vi "impedenzimetro.vi"() -> ()   [LabVIEW 2018]
uses:
  <vilib>/Analysis/4window.llb/windowTd.ctl
  <vilib>/Analysis/1siggen.llb/Ramp Pattern by Samples.vi
  <vilib>/DAQmx/write.llb/DAQmx Write (Analog Wfm 1Chan NSamp).vi
  <vilib>/DAQmx/create/channels.llb/DAQmx Create Channel (AO-Voltage-Basic).vi
  <vilib>/DAQmx/configure/timing.llb/DAQmx Timing (Sample Clock).vi
  <vilib>/DAQmx/miscellaneous.llb/DAQmx Fill In Error Info.vi
  <vilib>/measure/maspectr.llb/FFT Spectrum (Mag-Phase) for N Chan.vi
  <vilib>/DAQmx/read.llb/DAQmx Read (Analog 1D Wfm NChan NSamp).vi
  <resource>/objmgr/daqmx.rc
  <vilib>/measure/NI_MAPro.lvlib
  <vilib>/measure/NI_MABase.lvlib
  <vilib>/Analysis/NI_AALBase.lvlib
  <vilib>/Analysis/NI_AALPro.lvlib
panel:
  out "Zx":cdb=3019.4604118764787-15314.276810560117i
  in  "window":T1 items=["Rectangle"=0, "Hanning"=1, "Hamming"=2, "Blackman-Harris"=3, "Exact Blackman"=4, "Blackman"=5, "Flat Top"=6, "4 Term B-Harris "=7, "7 Term B-Harris"=8, "Low Sidelobe"=9, "Blackman Nuttall"=11, "Triangle"=30, "Bartlett-Hanning"=31, "Bohman"=32, "Parzen"=33, "Welch"=34, "Kaiser"=60, "Dolph-Chebyshev"=61, "Gaussian"=62]
  in  "amplitude[V]":dbl=10.0 format="%0.2p"
  in  "end[Hz]":dbl=1000.0 format="%0.2f"
  in  "start[Hz]":dbl=500.0 format="%0.2f"
  in  "samples":i32=10
  in  "Number of Samples":i32=20000
  in  "Sample Rate in[Hz]":dbl=200000.0 format="%#_13g"
  out "C[Farad]":dbl=1.039258628145917e-08 format="%#_6p"
  out "R[Ohm]":dbl=3019.4604118764787
  in  "R Shunt[Ohm]":dbl=300.0
  out "input":waveform(dbl)[](graph)=[{"t0"=timestamp(3731482242.5200343 s since 1904-01-01), "dt"=4.999999999999959e-06, "Y"=array[20000 elements], "attributes"=variant("NI_ChannelName"=variant(string "PXIe_NI6341/ai0"), "NI_UnitDescription"=variant(string "Volts"))}, {"t0"=timestamp(3731482242.520037 s since 1904-01-01), "dt"=4.999999999999959e-06, "Y"=array[20000 elements], "attributes"=variant("NI_ChannelName"=variant(string "PXIe_NI6341/ai1"), "NI_UnitDescription"=variant(string "Volts"))}]
  in  "Max Voltage in":dbl=10.0
  in  "Min Voltage out":dbl=-10.0
  in  "Input":tag="PXIe_NI6341/ai0:1"
  in  "Sample Rate out[Hz]":dbl=200000.0
  in  "Max Voltage out":dbl=10.0
  in  "Min Voltage out":dbl=-10.0
  out "Actual Sample Rate":dbl=200000.0 format="%0.2f"
  in  "Output":tag="PXIe_NI6341/ao0"
  in  "Configurazione scelta":string(combo)="serie"
  # "GENERAZIONE"
  # "CALCOLO DELLE COMPONENTI"
  # "ACQUISIZIONE"
  # "FREQUENZE"
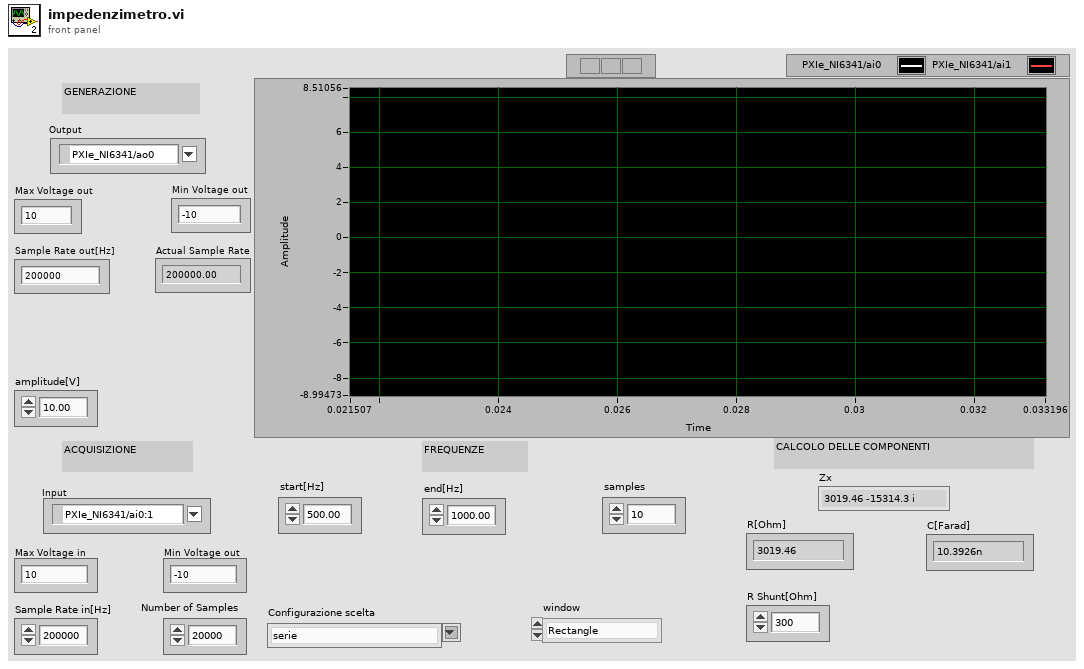
[diagram p1: front panel]
types:
  T1 = typedef "NI_AALPro.lvlib/windowTd.ctl" = u32
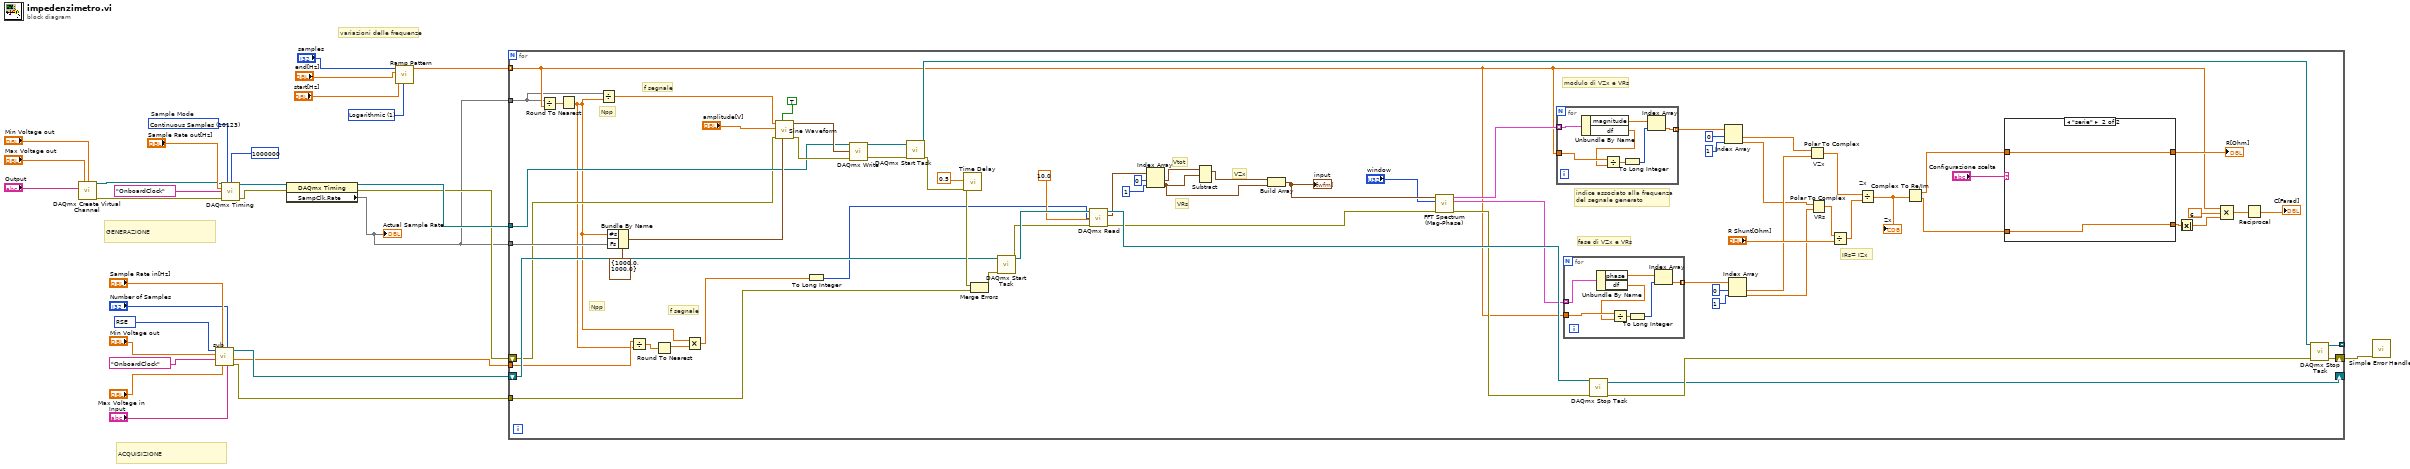
[diagram p0: block diagram]
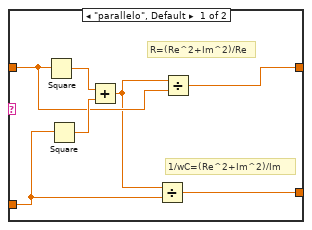
[diagram p2: hidden frame]
diagram:
  w3 = 10083 items=["default"=-1, "RSE"=10083, "NRSE"=10078, "Differential"=10106, "Pseudodifferential"=12529] ("Terminal Configuration")
  w9 = u16 1 items=["Linear", "Logarithmic"] ("type")
  w18 = 10123 items=["Finite Samples"=10178, "Continuous Samples"=10123, "Hardware Timed Single Point"=12522]  # Sample Mode
  # "ACQUISIZIONE"
  # "variazioni delle frequenze"
  # "GENERAZIONE"
  n1 = call-poly <vilib>:"DAQmx Create Virtual Channel.vi"("maximum value"="Max Voltage out", "minimum value"="Min Voltage out", "physical channels"="Output") -> ("task out"=w20:refnum<k21>, "error out"=w19:errorcluster)  [unwired: 11 in]
  n2 = call "sub.vi"("Physical Channel"="Input", "Number of Samples in"="Number of Samples", "Max Voltage"="Max Voltage in", "Sample Rate"="Sample Rate in[Hz]", "Sample Clock Source"=tag "OnboardClock", "Min Voltage"="Min Voltage out", "Terminal Configuration"=w3) -> ("error out"=w11:errorcluster, "Actual Sample Rate"=w1:dbl, "Refnum out"=w4:refnum<k21>)  [unwired: 1 in, 1 out]
  n3 = call-poly <vilib>:"DAQmx Timing.vi"("task/channels in"=w20, "sample mode"=w18, "samples per channel"=1000000, "rate"="Sample Rate out[Hz]", "source"=tag "OnboardClock" ("Sample Clock Source"), "error in"=w19) -> ("task out"=w16:refnum<k21>, "error out"=w17:errorcluster)  [unwired: 8 in]
  n4 = property class="DAQmx Timing"(reference=w16, error in=w17) -> (reference out=w15:refnum<k21>, error out=w12:errorcluster, "SampClk.Rate"=w2)
  "Actual Sample Rate" <- w2
  n5 = call-poly <vilib>:"Ramp Pattern.vi"("type"=w9, "start"="start[Hz]", "end"="end[Hz]", "samples"="samples") -> ("Ramp Pattern"=w6:dbl[])  [unwired: 6 in, 1 out]
  n6 = for {
    tunnel: [w85] -> _ mode=indexing
    shift-right: [w89] -> _
    shift-left: w4 -> [w84]
    tunnel: w6 -> [w40] mode=indexing
    tunnel: w11 -> [w83]
    tunnel: w15 -> [w82]
    tunnel: w2 -> [w81]
    shift-right: [w92] -> w13
    shift-left: w12 -> [w55]
    tunnel: w2 -> [w38]
    tunnel: w1 -> [w32]
    # "Npp"
    # "f segnale"
    # "indice associato alla frequenza\ndel segnale generato"
    # "f segnale"
    # "Npp"
    # "IRs= IZx"
    # "fase di VZx e VRs"
    # "modulo di VZx e VRs"
    # "VZx"
    # "VRs"
    # "Vtot"
    n7 = Divide(x=w38, y=w40) -> (x/y=w39:dbl)
    n8 = Round To Nearest(number=w39) -> (nearest integer value=w31:dbl)
    n9 = Divide(x=w38, y=w31) -> (x/y=w37:dbl)
    n10 = Bundle By Name(cluster=cluster{"Fs":dbl, "#s":dbl} {"Fs"=1000.0, "#s"=1000.0} ("sampling info"), "#s"=w31, "Fs"=w81) -> (w101:cluster{"Fs":dbl, "#s":dbl})
    n11 = Divide(x=w32, y=w31) -> (x/y=w36:dbl)
    n12 = Round To Nearest(number=w36) -> (nearest integer value=w35:dbl)
    n13 = Multiply(x=w31, y=w35) -> (x*y=w34:dbl)
    n14 = call <vilib>:"Sine Waveform.vi"("sampling info"=w101, "reset signal"=TRUE, "error in (no error)"=w55, "amplitude"="amplitude[V]", "frequency"=w37) -> ("error out"=w99:errorcluster, "signal out"=w98:waveform(dbl))  [unwired: 5 in]
    n15 = To Long Integer(number=w34) -> (32bit integer=w33:i32)
    n16 = call-poly <vilib>:"DAQmx Write.vi"("task/channels in"=w82, "data"=w98, "error in"=w99) -> ("task out"=w100:refnum<k21>, "error out"=w97:errorcluster)  [unwired: 10 in, 1 out]
    n17 = call <vilib>:"DAQmx Start Task.vi"("task/channels in"=w100, "error in"=w97) -> ("task out"=w96:refnum<k21>, "error out"=w93:errorcluster)  [unwired: 12 in]
    n18 = call "Time Delay"("error in (no error)"=w93, "Delay Time (s)"=0.5) -> ("error out"=w87:errorcluster)  [unwired: 9 in]
    n19 = Merge Errors(w87, w83) -> (w88:errorcluster)
    n20 = call <vilib>:"DAQmx Start Task.vi"("task/channels in"=w84, "error in"=w88) -> ("task out"=w95:refnum<k21>, "error out"=w94:errorcluster)  [unwired: 12 in]
    n21 = call-poly <vilib>:"DAQmx Read.vi"("task/channels in"=w95, "number of samples per channel"=w33, "timeout"=10.0, "error in"=w94) -> ("task out"=w91:refnum<k21>, "data"=w49:waveform(dbl)[], "error out"=w65:errorcluster)  [unwired: 9 in]
    n22 = Index Array(array=w49, index #1=0 ("index"), index #2=1 ("index")) -> (element #1=w48:waveform(dbl), element #2=w42:waveform(dbl))
    n23 = Subtract(1:w42, 2:w48) -> (0:w45:waveform(dbl))  [unwired: 1 in, 1 out]
    n24 = Build Array(w45, w42) -> (w44:waveform(dbl)[])
    "input" <- w44
    n25 = call-poly <vilib>:"FFT Spectrum (Mag-Phase).vi"("error in (no error)"=w65, "window"="window", "time signals"=w44) -> ("error out"=w74:errorcluster, "phases"=w76:cluster{"f0":dbl, "df":dbl, "phase":dbl[]}[], "magnitudes"=w75:cluster{"f0":dbl, "df":dbl, "magnitude":dbl[]}[])  [unwired: 4 in, 2 out]
    n26 = for {
      tunnel: w75 -> [w124] mode=indexing
      tunnel: [w123] -> w71 mode=indexing
      tunnel: w40 -> [w122]
      n27 = Unbundle By Name(w124) -> ("magnitude"=w125:dbl[], "df"=w121:dbl)
      n28 = Divide(x=w122, y=w121) -> (x/y=w120:dbl)
      n29 = To Long Integer(number=w120) -> (32bit integer=w119:i32)
      n30 = Index Array(array=w125, index=w119) -> (element=w123:dbl)
    }
    n31 = for {
      tunnel: w76 -> [w117] mode=indexing
      tunnel: [w116] -> w77 mode=indexing
      tunnel: w40 -> [w115]
      n32 = Unbundle By Name(w117) -> ("phase"=w118:dbl[], "df"=w114:dbl)
      n33 = Divide(x=w115, y=w114) -> (x/y=w113:dbl)
      n34 = To Long Integer(number=w113) -> (32bit integer=w112:i32)
      n35 = Index Array(array=w118, index=w112) -> (element=w116:dbl)
    }
    n36 = call <vilib>:"DAQmx Stop Task.vi"("task/channels in"=w91, "error in"=w74) -> ("task out"=w89:refnum<k21>, "error out"=w90:errorcluster)  [unwired: 12 in]
    n37 = Index Array(array=w71, index #1=0 ("index"), index #2=1 ("index")) -> (element #1=w64:dbl, element #2=w58:dbl)
    n38 = Index Array(array=w77, index #1=0 ("index"), index #2=1 ("index")) -> (element #1=w63:dbl, element #2=w57:dbl)
    n39 = Polar To Complex "VZx"(1:w63, 2:w64) -> (0:w56:cdb)
    n40 = Polar To Complex "VRs"(1:w57, 2:w58) -> (0:w52:cdb)
    n41 = Divide(x=w52, y="R Shunt[Ohm]") -> (x/y=w51:cdb)
    n42 = Divide "Zx"(x=w56, y=w51) -> (x/y=w62:cdb)
    "Zx" <- w62
    n43 = Complex To Re/Im(x + iy=w62) -> (x=w61:dbl, y=w60:dbl)
    n44 = case shown="\"serie\"" "Configurazione scelta" {
      tunnel: w61 -> [w106 w111]
      tunnel: w60 -> [w107 w110]
      tunnel: [w105 w111] -> w68
      tunnel: [w104 w110] -> w54
      frame "parallelo", Default {
        # "1/wC=(Re^2+Im^2)/Im"
        # "R=(Re^2+Im^2)/Re"
        n45 = Square(x=w106) -> (x^2=w109:dbl)
        n46 = Square(x=w107) -> (x^2=w108:dbl)
        n47 = Add(x=w109, y=w108) -> (x+y=w103:dbl)
        n48 = Divide(x=w103, y=w107) -> (x/y=w104:dbl)
        n49 = Divide(x=w103, y=w106) -> (x/y=w105:dbl)
      }
      frame "serie" {
      }
    }
    "R[Ohm]" <- w68
    n50 = Absolute Value(x=w54) -> (abs(x)=w50:dbl)
    n51 = Compound Arithmetic op=MULTIPLY(w40, 6.283185307179586, w50) -> (w67:dbl)
    n52 = Reciprocal(x=w67) -> (1/x=→"C[Farad]":dbl)
    n53 = call <vilib>:"DAQmx Stop Task.vi"("task/channels in"=w96, "error in"=w90) -> ("task out"=w85:refnum<k21>, "error out"=w92:errorcluster)  [unwired: 12 in]
  }
  n54 = call <vilib>:"Simple Error Handler.vi"("error in (no error)"=w13) -> ()  [unwired: 4 in, 5 out]
